vi "ZSliceCompute.vi"(9 "Function":T1, 10 "Optimise Objective position":bool, 11 "ZStack (um)":cluster{"Zstart":dbl, "Zstop":dbl, "Zstep":dbl}) -> (1 "# of Z-planes":i32, 2 "AOL Z Planes(um)":dbl[](array[numeric]) format="%#_12f", 3 "Motor Z Planes(um)":dbl[](array[numeric]) format="%#_12f", 5 "ZStack (um)":cluster{"Zstart":dbl, "Zstop":dbl, "Zstep":dbl})   [LabVIEW 2020]
uses:
  Typedefs/Read Write Enum.ctl
  Global Variables/General Globals.vi
panel:
  # "SUBROUTINE"
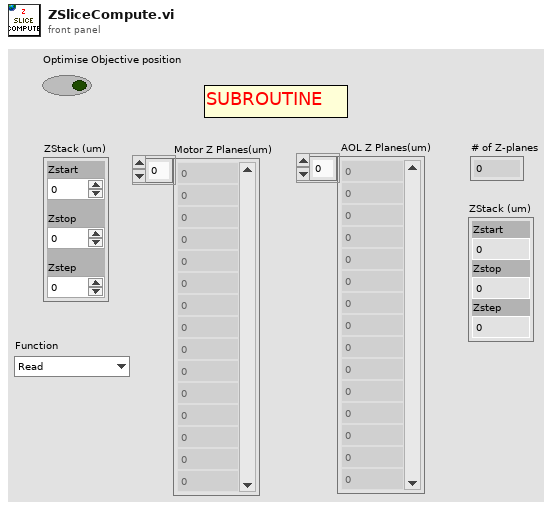
[diagram p1: front panel]
types:
  T1 = typedef "Read Write Enum.ctl" = enum16{"Read", "Write"}
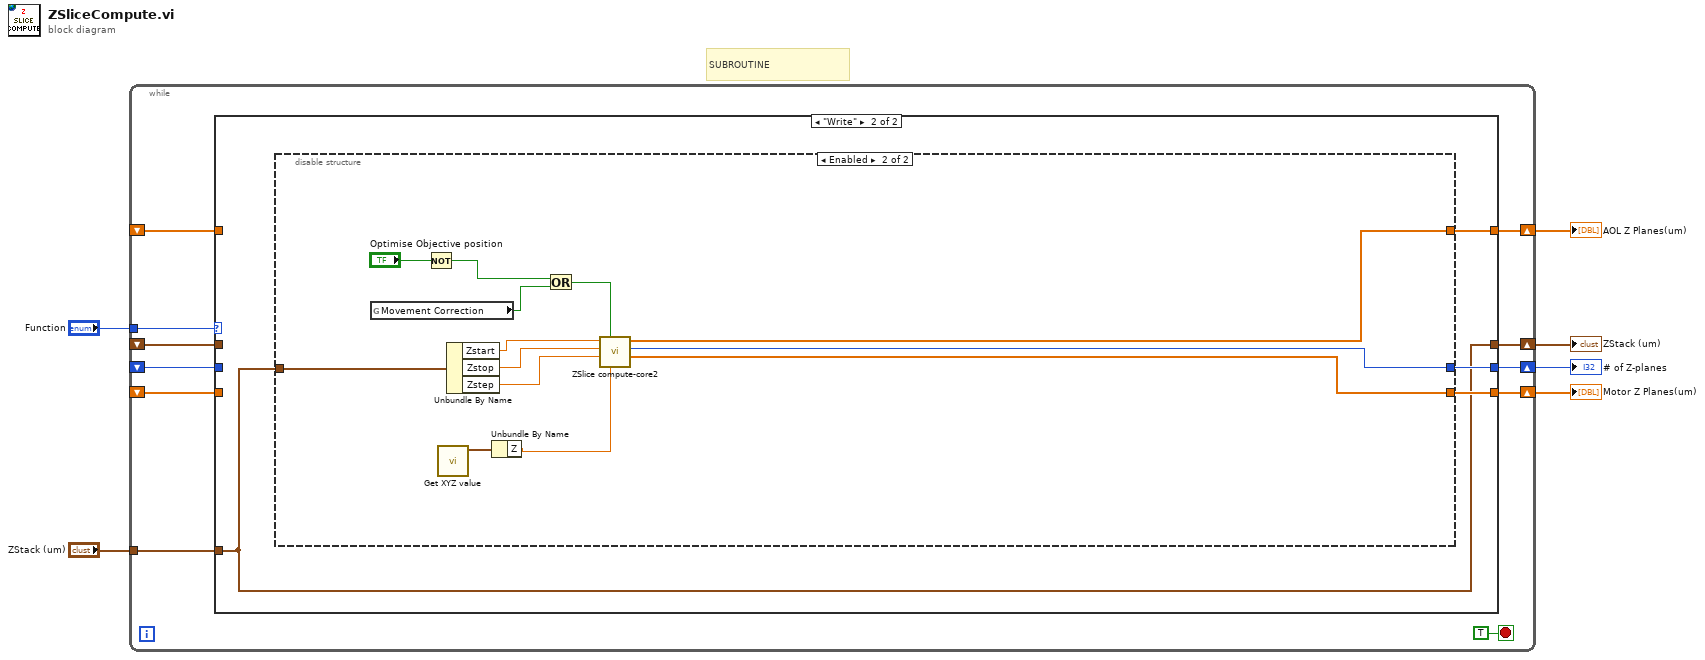
[diagram p0: block diagram]
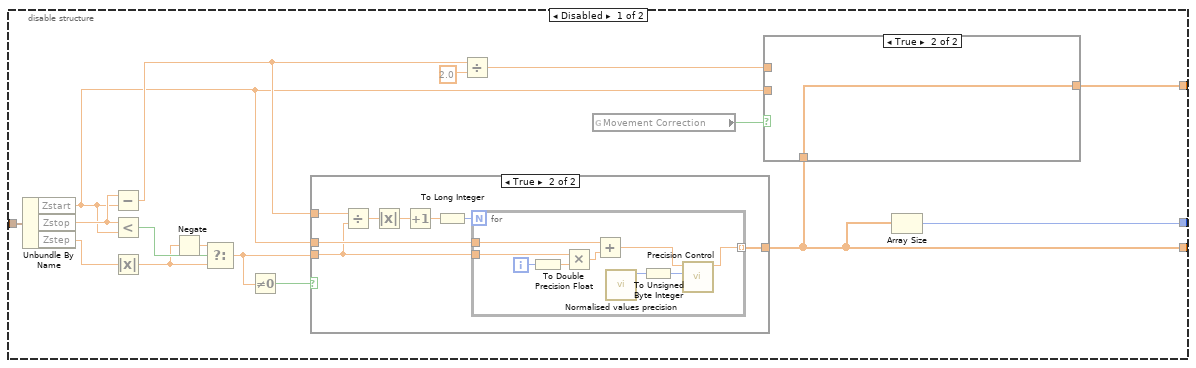
[diagram p3: hidden frame]
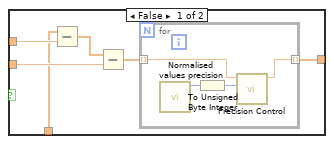
[diagram p4: hidden frame]
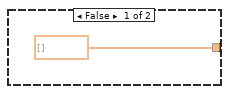
[diagram p5: hidden frame]
diagram:
  # "SUBROUTINE"
  n1 = while {
    shift-right: [w15] -> w5
    shift-left: _ -> [w10]
    shift-right: [w16] -> w6
    shift-left: _ -> [w11]
    shift-right: [w14] -> w4
    shift-left: _ -> [w12]
    tunnel: "Function" -> [w9]
    shift-right: [w8] -> w1
    shift-left: _ -> [w17]
    tunnel: "ZStack (um)" -> [w7]
    stop <- TRUE stop-if-true
    n2 = case shown="\"Write\"" w9 {
      tunnel: w17 -> [w18 _]
      tunnel: [w20 w25] -> w16
      tunnel: [w19 w24] -> w15
      tunnel: [w21 w23] -> w14
      tunnel: w12 -> [w21 _]
      tunnel: w11 -> [w20 _]
      tunnel: w10 -> [w19 _]
      tunnel: [w18 w22] -> w8
      tunnel: w7 -> [_ w22]
      frame "Read", Default {
      }
      frame "Write" {
        n3 = disable-structure shown="Enabled" {
          disable-tunnel: [w30 w78] -> w25
          disable-tunnel: [w29 w77] -> w24
          disable-tunnel: [w28 w79] -> w23
          disable-tunnel: w22 -> [w27 w83]
          frame Disabled {
            n4 = Unbundle By Name(w27) -> ("Zstart"=w31:dbl, "Zstop"=w38:dbl, "Zstep"=w37:dbl)
            n5 = Subtract(x=w38, y=w31) -> (x-y=w34:dbl)
            n6 = Less?(x=w38, y=w31) -> (x < y?=w41:bool)
            n7 = Absolute Value(x=w37) -> (abs(x)=w39:dbl)
            n8 = Negate(x=w39) -> (-x=w40:dbl)
            n9 = Select(t=w40, s=w41, f=w39) -> (s? t:f=w36:dbl)
            n10 = Not Equal To 0?(x=w36) -> (x != 0?=w35:bool)
            n11 = case shown="True" w35 {
              tunnel: w34 -> [_ w61]
              tunnel: w31 -> [_ w57]
              tunnel: w36 -> [_ w56]
              tunnel: [dbl[] [] w55] -> w29
              frame False {
              }
              frame True {
                n12 = Divide(x=w61, y=w56) -> (x/y=w58:dbl)
                n13 = Absolute Value(x=w58) -> (abs(x)=w59:dbl)
                n14 = Increment(x=w59) -> (x+1=w60:dbl)
                n15 = To Long Integer(number=w60) -> (32bit integer=w54:i32)
                n16 = for {
                  N: w54 -> [_]
                  tunnel: w56 -> [w69]
                  tunnel: w57 -> [w68]
                  tunnel: [w62] -> w55 mode=indexing
                  i -> [w70]
                  n17 = To Double Precision Float(number=w70) -> (double precision float=w66:dbl)
                  n18 = Multiply(x=w69, y=w66) -> (x*y=w67:dbl)
                  n19 = Add(x=w68, y=w67) -> (x+y=w63:dbl)
                  n20 = call "Normalised values precision.vi"() -> ("Normalised values precision"=w64:i32)  [unwired: 11 in]
                  n21 = To Unsigned Byte Integer(number=w64) -> (unsigned 8bit integer=w65:u8)
                  n22 = call <userlib>:"Precision Control.vi"("Precision"=w65, "Input Value"=w63) -> ("Output Value"=w62:dbl)  [unwired: 8 in, 1 out]
                }
              }
            }
            n23 = Divide(x=w34, y=2.0) -> (x/y=w32:dbl)
            n24 = global read "General Globals.vi" "Movement Correction"() -> (w26:bool)
            n25 = case shown="True" w26 {
              tunnel: w32 -> [w46 _]
              tunnel: w31 -> [w45 _]
              tunnel: w29 -> [w44 w52]
              tunnel: [w42 w52] -> w28
              frame False {
                n26 = Subtract(x=w44, y=w46) -> (x-y=w47:dbl[])
                n27 = Subtract(x=w47, y=w45) -> (x-y=w43:dbl[])
                n28 = for {
                  tunnel: [w49] -> w42 mode=indexing
                  tunnel: w43 -> [w48] mode=indexing
                  n29 = call "Normalised values precision.vi"() -> ("Normalised values precision"=w50:i32)  [unwired: 11 in]
                  n30 = To Unsigned Byte Integer(number=w50) -> (unsigned 8bit integer=w51:u8)
                  n31 = call <userlib>:"Precision Control.vi"("Precision"=w51, "Input Value"=w48) -> ("Output Value"=w49:dbl)  [unwired: 8 in, 1 out]
                }
              }
              frame True {
              }
            }
            n32 = Array Size(array=w29) -> (size(s)=w30:i32)
          }
          frame Enabled {
            n33 = global read "General Globals.vi" "Movement Correction"() -> (w72:bool)
            n34 = Not(x="Optimise Objective position") -> (.not. x?=w73:bool)
            n35 = call "Get XYZ value.vi"() -> ("Stage XYZ Position"=w76:cluster{"X":sgl, "Y":sgl, "Z":sgl})  [unwired: 11 in]
            n36 = Unbundle By Name(w83) -> ("Zstart"=w82:dbl, "Zstop"=w81:dbl, "Zstep"=w80:dbl)
            n37 = Unbundle By Name(w76) -> ("Z"=w75:sgl)
            n38 = Or(x=w73, y=w72) -> (x .or. y?=w71:bool)
            n39 = call "ZSlice compute-core2.vi"("ZStage Pos"=w75, "Objective Pos Locked"=w71, "ZStep"=w80, "ZStop"=w81, "ZStart"=w82) -> ("Motor Z Planes(um)"=w77:dbl[], "# of Z-planes"=w78:i32, "AOL Z Planes(um)"=w79:dbl[])  [unwired: 2 in, 2 out]
          }
        }
      }
    }
  }
  "Motor Z Planes(um)" <- w5
  "AOL Z Planes(um)" <- w4
  "# of Z-planes" <- w6
  "ZStack (um)" <- w1
